vi "matrix.vi"(0 "Horizon":i32, 5 "A":dbl[](array[numeric]), 7 "X * Y in":dbl[](array[numeric]), 9 "Real Matrix (Column Vector)":T1, 12 "Numeric":i32) -> (2 "Inverse Matrix":T1, 3 "Real Matrix":T1, 4 "n":i32, 6 "m":i32, 8 "new element/subarray":dbl, 10 "X * Y out":dbl[](array[numeric]), 13 "A * B":T1, 14 "A * B 2":T1)   [LabVIEW 2016]
uses:
  <vilib>/Analysis/Matrix/Datatypes/RealMatrix.ctl
  <vilib>/Analysis/2dsp.llb/1D Convolution (DBL).vi
  <vilib>/Analysis/7linalg.llb/Create Special Real Matrix.vi
  <vilib>/Analysis/Matrix/Numeric/Conversions/Array To Matrix - RA2.vi
  <vilib>/Analysis/Matrix/Numeric/Conversions/Array To Matrix - RA.vi
  <vilib>/Analysis/baseanly.llb/Real Inverse Matrix.vi
  <vilib>/Analysis/Matrix/Numeric/Multiply/Multiply - RM,RM.vi
  <vilib>/Analysis/NI_AALPro.lvlib
  <vilib>/Analysis/Matrix/NI_Matrix.lvlib
  <vilib>/Analysis/NI_AALBase.lvlib
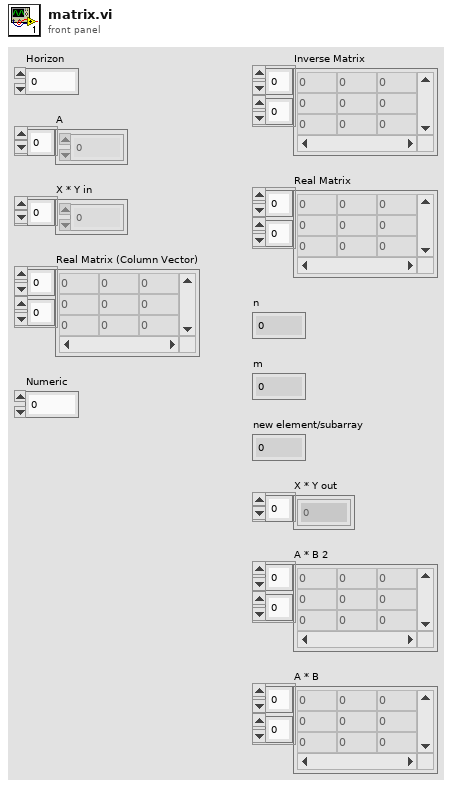
[diagram p1: front panel]
types:
  T1 = typedef "NI_Matrix.lvlib/RealMatrix.ctl" = dbl[][]
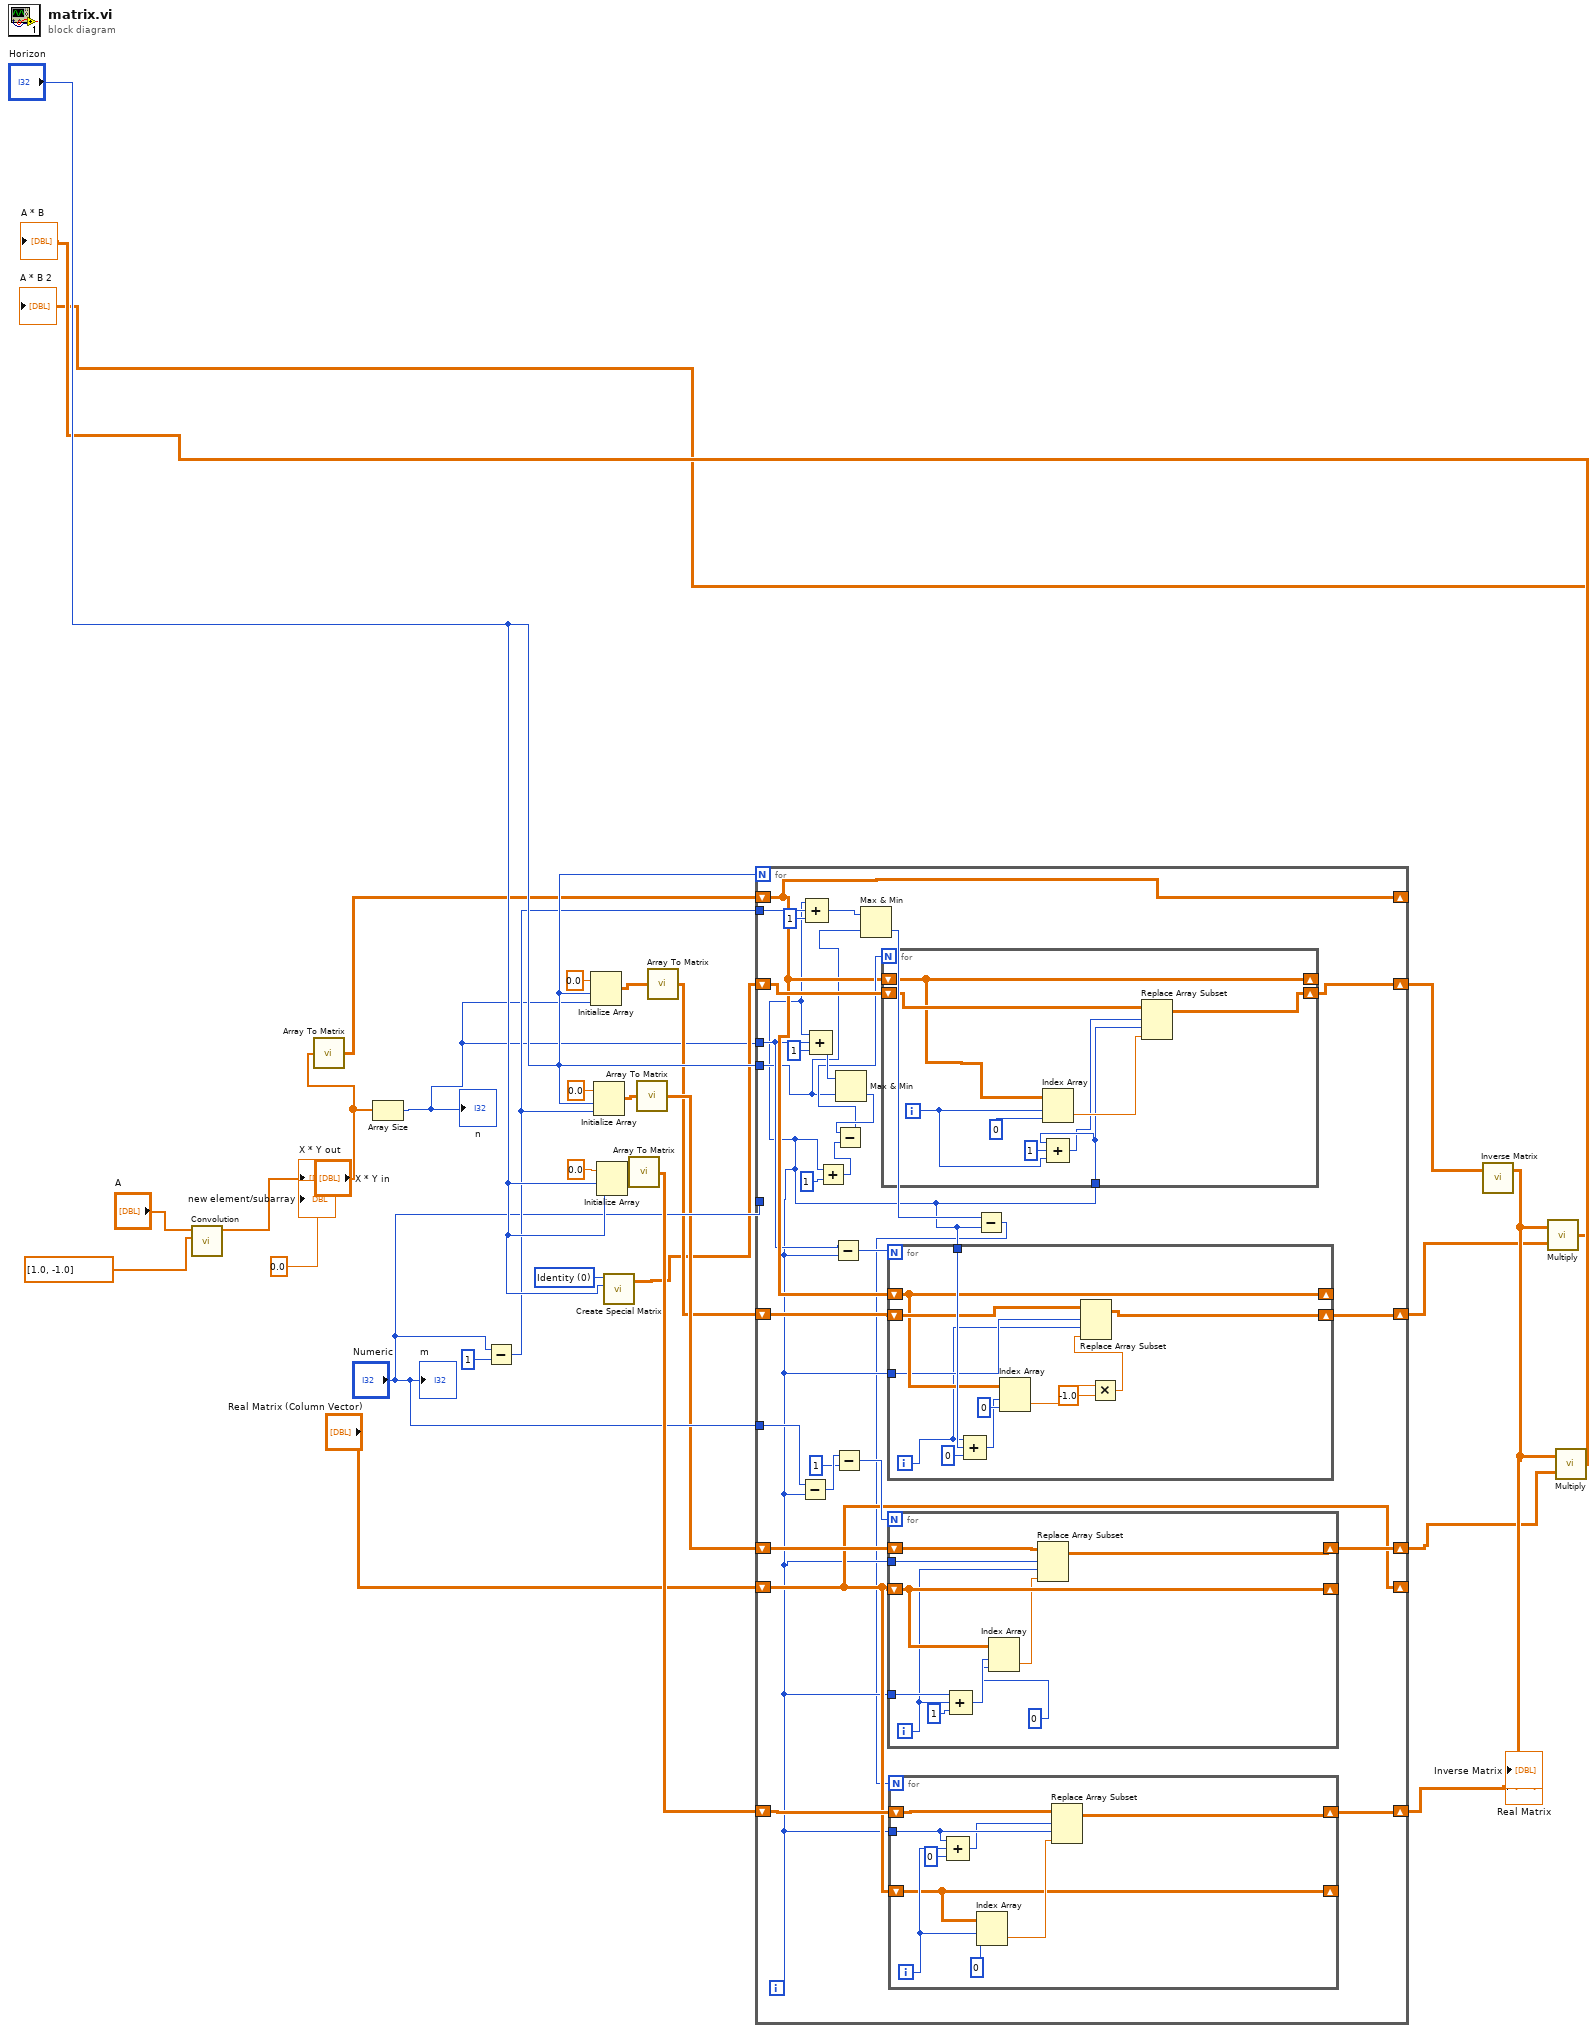
[diagram p0: block diagram]
diagram:
  w8 = 0 items=["Identity", "Diagonal", "Toeplitz", "Vandermonde", "Companion", "Hankel", "Hadamard", "Wilkinson", "Hilbert", "Inverse Hilbert", "Rosser", "Pascal"] ("matrix type")
  n1 = call-poly <vilib>:"Convolution.vi"("Y"=dbl[] [1.0, -1.0] ("A 2"), "X"="A") -> ("X * Y"=→"X * Y out":dbl[])  [unwired: 8 in, 1 out]
  n2 = call-poly <vilib>:"Array To Matrix.vi"("Real 1D Array"="X * Y in") -> ("Real Matrix (Column Vector)"=w13:T1)
  n3 = Array Size(array="X * Y in") -> (size(s)=w15:i32)
  "n" <- w15
  n4 = Subtract(x="Numeric", y=1) -> (x-y=w22:i32)
  n5 = Initialize Array(0.0 ("element"), "Horizon", w15) -> (w9:dbl[][])
  n6 = Initialize Array(0.0 ("element"), "Horizon", w22) -> (w10:dbl[][])
  n7 = Initialize Array(0.0 ("element"), "Horizon", "Horizon") -> (w11:dbl[][])
  n8 = call-poly <vilib>:"Create Special Matrix.vi"("matrix type"=w8, "matrix size"="Horizon") -> ("Special Matrix"=w16:T1)  [unwired: 3 in, 1 out]
  n9 = call-poly <vilib>:"Array To Matrix.vi"("Real 2D Array"=w11) -> ("Real Matrix"=w21:T1)
  n10 = call-poly <vilib>:"Array To Matrix.vi"("Real 2D Array"=w10) -> ("Real Matrix"=w18:T1)
  n11 = call-poly <vilib>:"Array To Matrix.vi"("Real 2D Array"=w9) -> ("Real Matrix"=w17:T1)
  n12 = for {
    N: "Horizon" -> [_]
    shift-right: [w58] -> w23
    shift-left: w16 -> [w59]
    shift-right: [w49] -> _
    shift-left: w13 -> [w49]
    tunnel: "Numeric" -> [_]
    tunnel: w15 -> [w48]
    tunnel: "Horizon" -> [w37]
    shift-right: [w50] -> w24
    shift-left: w17 -> [w51]
    shift-right: [w45] -> w25
    shift-left: w18 -> [w46]
    shift-right: [w38] -> _
    shift-left: "Real Matrix (Column Vector)" -> [w38]
    tunnel: "Numeric" -> [w44]
    shift-right: [w39] -> w26
    shift-left: w21 -> [w40]
    tunnel: w22 -> [w35]
    i -> [w32]
    n13 = Subtract(x=w44, y=w32) -> (x-y=w43:i32)
    n14 = Compound Arithmetic op=ADD(w32, w35, 1 ("value")) -> (w36:i32)
    n15 = Compound Arithmetic op=ADD(w32, w48, 1 ("value")) -> (w56:i32)
    n16 = Add(x=w32, y=1) -> (x+y=w53:i32)
    n17 = Subtract(x=w48, y=w32) -> (x-y=w47:i32)
    n18 = Subtract(x=w43, y=1) -> (x-y=w41:i32)
    n19 = Max & Min(x=w56, y=w37) -> (min(x,y)=w55:i32)  [unwired: 1 out]
    n20 = Subtract(x=w55, y=w53) -> (x-y=w52:i32)
    n21 = Max & Min(x=w36, y=w37) -> (min(x,y)=w33:i32)  [unwired: 1 out]
    n22 = for {
      N: w52 -> [_]
      shift-right: [w98] -> w58
      shift-left: w59 -> [w99]
      tunnel: w32 -> [w94]
      shift-right: [w97] -> _
      shift-left: w49 -> [w97]
      i -> [w92]
      n23 = Index Array(array=w97, index (row)=w92, index (col)=0 ("index (row)")) -> (element=w95:dbl)
      n24 = Compound Arithmetic op=ADD(w94, 1 ("value"), w92) -> (w91:i32)
      n25 = Replace Array Subset(array=w99, new element=w95, index (row)=w91, index (col)=w94) -> (w98:T1)
    }
    n26 = for {
      N: w47 -> [_]
      shift-right: [w85] -> w50
      shift-left: w51 -> [w86]
      shift-right: [w84] -> _
      shift-left: w49 -> [w84]
      tunnel: w32 -> [w89]
      tunnel: w32 -> [w83]
      i -> [w82]
      n27 = Compound Arithmetic op=ADD(w82, w89, 0 ("value")) -> (w87:i32)
      n28 = Index Array(array=w84, index (row)=w87, index (col)=0) -> (element=w80:dbl)
      n29 = Multiply(x=w80, y=-1.0) -> (x*y=w79:dbl)
      n30 = Replace Array Subset(array=w86, new element=w79, index (row)=w83, index (col)=w82) -> (w85:T1)
    }
    n31 = for {
      N: w41 -> [_]
      shift-right: [w76] -> w45
      shift-left: w46 -> [w77]
      shift-right: [w78] -> _
      shift-left: w38 -> [w78]
      tunnel: w32 -> [w74]
      tunnel: w32 -> [w72]
      i -> [w71]
      n32 = Compound Arithmetic op=ADD(w74, w71, 1 ("value")) -> (w70:i32)
      n33 = Index Array(array=w78, index (row)=w70, index (col)=0 ("index (row)")) -> (element=w73:dbl)
      n34 = Replace Array Subset(array=w77, new element=w73, index (row)=w72, index (col)=w71) -> (w76:T1)
    }
    n35 = Subtract(x=w33, y=w32) -> (x-y=w31:i32)
    n36 = for {
      N: w31 -> [_]
      shift-right: [w67] -> w39
      shift-left: w40 -> [w68]
      shift-right: [w60] -> _
      shift-left: w38 -> [w60]
      tunnel: w32 -> [w64]
      i -> [w63]
      n37 = Compound Arithmetic op=ADD(w64, w63, 0 ("value")) -> (w61:i32)
      n38 = Index Array(array=w60, index (row)=w63, index (col)=0) -> (element=w65:dbl)
      n39 = Replace Array Subset(array=w68, new element=w65, index (row)=w61, index (col)=w64) -> (w67:T1)
    }
  }
  "Real Matrix" <- w26
  n40 = call-poly <vilib>:"Inverse Matrix.vi"("Input Matrix"=w23) -> ("Inverse Matrix"=w27:T1)  [unwired: 1 in, 1 out]
  "Inverse Matrix" <- w27
  n41 = call-poly <vilib>:"Multiply.vi"("Real Matrix B"=w24, "Real Matrix A"=w27) -> ("A * B"=→"A * B 2":T1)
  n42 = call-poly <vilib>:"Multiply.vi"("Real Matrix B"=w25, "Real Matrix A"=w27) -> ("A * B"=→"A * B":T1)
  "m" <- "Numeric"
  "new element/subarray" <- 0.0 ("new element/subarray")
